vi "Sensifier.vi"(11 "Array":string[](array[string])) -> (1 "Removed Strings":string[](array[string]), 2 "Has Errors?":bool, 3 "Sensed":string[](array[string]))   [LabVIEW 2014]
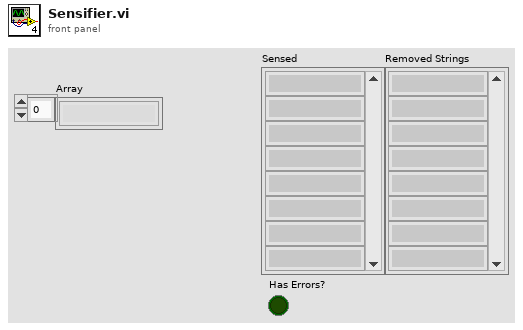
[diagram p1: front panel]
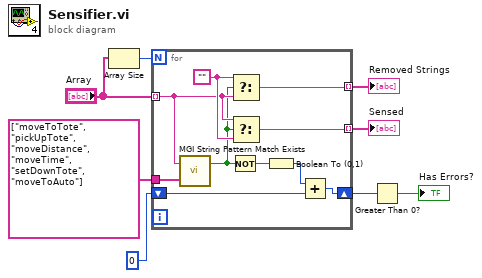
[diagram p0: block diagram]
diagram:
  n1 = Array Size(array="Array") -> (size(s)=w6:i32)
  n2 = for {
    N: w6 -> [_]
    tunnel: "Array" -> [w12] mode=indexing
    tunnel: string[] ["moveToTote", "pickUpTote", "moveDistance", "moveTime", "setDownTote", "moveToAuto"] ("string array") -> [w18]
    tunnel: [w17] -> w1 mode=indexing
    shift-right: [w16] -> w5
    shift-left: i16 0 -> [w15]
    tunnel: [w11] -> w3 mode=indexing
    w13 = ""
    n3 = call <userlib>:"MGI String Pattern Match Exists.vi"("Patterns to Try"=w18, "String"=w12) -> ("Match Found"=w9:bool)  [unwired: 1 out]
    n4 = Not(x=w9) -> (.not. x?=w10:bool)
    n5 = Select(t=w13, s=w9, f=w12) -> (s? t:f=w11:string)
    n6 = Select(t=w12, s=w9, f=w13) -> (s? t:f=w17:string)
    n7 = Boolean To (0,1)(Boolean=w10) -> (0, 1=w14:i16)
    n8 = Add(x=w14, y=w15) -> (x+y=w16:i16)
  }
  "Sensed" <- w1
  "Removed Strings" <- w3
  n9 = Greater Than 0?(x=w5) -> (x > 0?=→"Has Errors?":bool)
